vi "HTML Report Labeled String Table.vi"(2 "column width (100)":dbl=100.0, 4 "Show Grid":bool, 5 "width":string, 6 "align (default)":T1, 7 "transpose array (F)":bool, 8 "row headers":string[](array[string]), 9 "column headers":string[](array[string]), 10 "table contents":string[][](array[string]), 11 "HTML in":string) -> (3 "HTML out":string)   [LabVIEW 2020, in "NI_ReportGenerationCore.lvlib"]
doc: "Constructs HTML code to describe a table containing table contents, row headers and column headers."
uses:
  <vilib>/Utility/NIReport.llb/NI_ReportGenerationCore.lvlib
  <vilib>/Utility/NIReport.llb/HTML Report Text Alignment.ctl
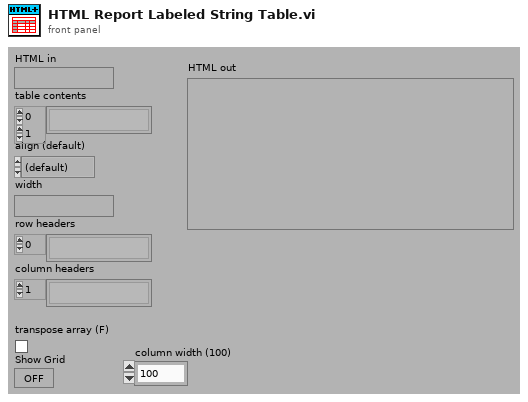
[diagram p1: front panel]
types:
  T1 = typedef "NI_ReportGenerationCore.lvlib/HTML Report Text Alignment.ctl" = enum16{"(default)", "LEFT", "CENTER", "RIGHT"}
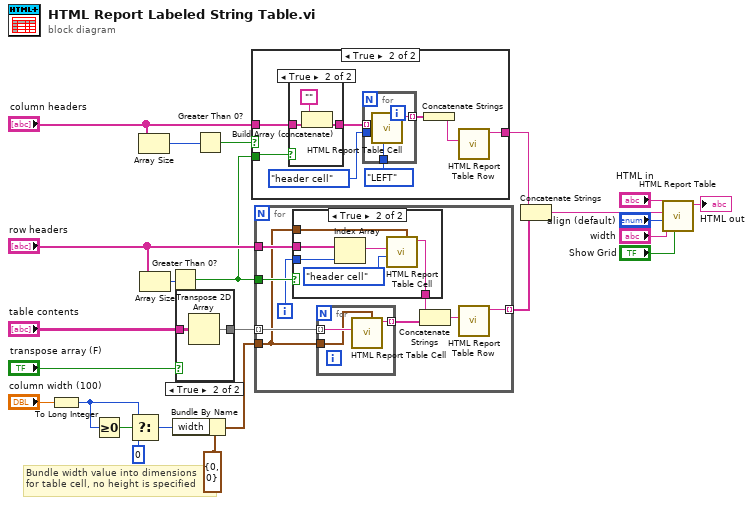
[diagram p0: block diagram]
diagram:
  # "Bundle width value into dimensions\nfor table cell, no height is specified"
  n1 = To Long Integer(number="column width (100)") -> (32bit integer=w3:i32)
  n2 = Greater Or Equal To 0?(x=w3) -> (x >= 0?=w4:bool)
  n3 = Select(t=w3, s=w4, f=0 ("32bit integer")) -> (s? t:f=w1:i32)
  n4 = Array Size(array="column headers") -> (size(s)=w16:i32)
  n5 = Array Size(array="row headers") -> (size(s)=w12:i32)
  n6 = Greater Than 0?(x=w12) -> (x > 0?=w10:bool)
  n7 = Bundle By Name(cluster=cluster{"height":i32, "width":i32} {"height"=0, "width"=0} ("pixel size (default)"), "width"=w1) -> (w5:cluster{"height":i32, "width":i32})
  n8 = case shown="True" "transpose array (F)" {
    tunnel: "table contents" -> [w25 w27]
    tunnel: [w25 w26] -> w17
    frame False {
    }
    frame True {
      n9 = Transpose 2D Array(2D array=w27) -> (transposed array=w26:string[][])
    }
  }
  n10 = Greater Than 0?(x=w16) -> (x > 0?=w14:bool)
  n11 = case shown="True" w14 {
    tunnel: "column headers" -> [_ w29]
    tunnel: [_ w32] -> w13
    tunnel: w10 -> [_ w31]
    frame False {
    }
    frame True {
      n12 = case shown="True" w31 {
        tunnel: w29 -> [w36 w39]
        tunnel: [w36 w38] -> w30
        frame False {
        }
        frame True {
          n13 = Build Array (concatenate)("" ("Empty String Constant"), w39) -> (w38:string[])
        }
      }
      n14 = for {
        tunnel: [w43] -> w35 mode=indexing
        tunnel: enum16{"data cell", "header cell"}."header cell" ("cell type (data cell)") -> [w42]
        tunnel: w30 -> [w41] mode=indexing
        tunnel: HTML_Report_Text_Alignment."LEFT" ("align (default)") -> [w40]
        n15 = call <vilib>:"HTML Report Table Cell.vi"("align (default)"=w40, "cell type (data cell)"=w42, "cell contents"=w41) -> ("table cells out"=w43:string)  [unwired: 1 in, 7 out]
      }
      n16 = Concatenate Strings(w35) -> (w33:string)
      n17 = call <vilib>:"HTML Report Table Row.vi"("table cells"=w33) -> ("table rows out"=w32:string)  [unwired: 1 in, 5 out]
    }
  }
  n18 = for {
    tunnel: w17 -> [w52] mode=indexing
    tunnel: [w49] -> w24 mode=indexing
    tunnel: w10 -> [w48]
    tunnel: "row headers" -> [w47]
    tunnel: w5 -> [w44]
    i -> [w46]
    n19 = case shown="True" w48 {
      tunnel: w47 -> [_ w58]
      tunnel: w46 -> [_ w57]
      tunnel: [_ w54] -> w45
      tunnel: w44 -> [_ w53]
      frame False {
      }
      frame True {
        n20 = Index Array(array=w58, index=w57) -> (element=w56:string)
        n21 = call <vilib>:"HTML Report Table Cell.vi"("pixel size (default)"=w53, "cell type (data cell)"=enum16{"data cell", "header cell"}."header cell", "cell contents"=w56) -> ("table cells out"=w54:string)  [unwired: 1 in, 7 out]
      }
    }
    n22 = for {
      tunnel: w52 -> [w60] mode=indexing
      tunnel: [w61] -> w51 mode=indexing
      tunnel: w44 -> [w59]
      n23 = call <vilib>:"HTML Report Table Cell.vi"("pixel size (default)"=w59, "cell contents"=w60) -> ("table cells out"=w61:string)  [unwired: 1 in, 8 out]
    }
    n24 = Concatenate Strings(w45, w51) -> (w50:string)
    n25 = call <vilib>:"HTML Report Table Row.vi"("table cells"=w50) -> ("table rows out"=w49:string)  [unwired: 1 in, 5 out]
  }
  n26 = Concatenate Strings(w13, w24) -> (w23:string)
  n27 = call <vilib>:"HTML Report Table.vi"("Show Grid"="Show Grid", "width"="width", "align (default)"="align (default)", "table rows"=w23, "HTML in"="HTML in") -> ("HTML out"=→"HTML out":string)  [unwired: 3 out]
